vi "Quick Start - Complete Streaming with Datasource Creation.vi"() -> ()   [LabVIEW 2020]
uses:
  Nominal Client/Nominal Client.lvclass/Nominal Client.ctl
  8bc873d6-11f2-47b8-afa9-2ee06eb45ce7.vi
  Nominal Client/private_data.set.vi
  <vilib>/Utility/file.llb/Application Directory.vi
  <vilib>/Utility/error.llb/Error Cluster From Error Code.vi
  submodules/reqwest-labview/lv-src/reqwest/create.vi
  Nominal Client/Palette Items/who_am_i.vi
  Nominal Client/asset.get.vi
  User/User.lvclass
  Nominal Client/Nominal Client.lvclass
  nominal types/workspace/workspace.lvclass
  submodules/reqwest-labview/lv-src/reqwest/reqwest.lvclass
  asset/asset.lvclass
  datasources/dataset/dataset.lvclass
  submodules/nominal-streaming-labview-ffi/lv_src/Stream/Stream.lvclass
  submodules/nominal-streaming-labview-ffi/lv_src/Channel/Channel.lvclass
panel:
  in  "API Token":string
  in  "Stop":bool
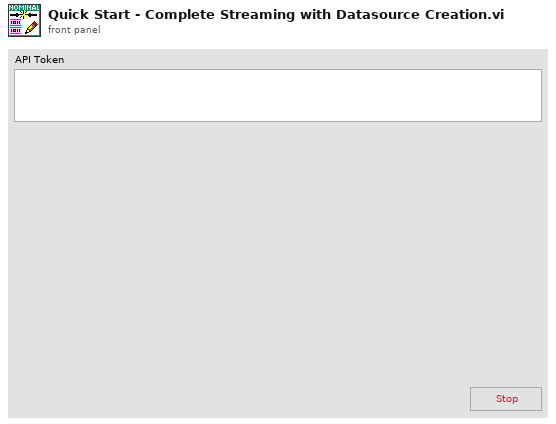
[diagram p1: front panel]
types:
  T1 = cluster{"channel":string, "current time":timestamp, "data":dbl}
  T2 = cluster{"[0]":refnum<queue>, "[1]":refnum<queue>, "[2]":refnum<queue>}
  T3 = cluster{"channel":string, "current time":timestamp, "data":dbl}[]
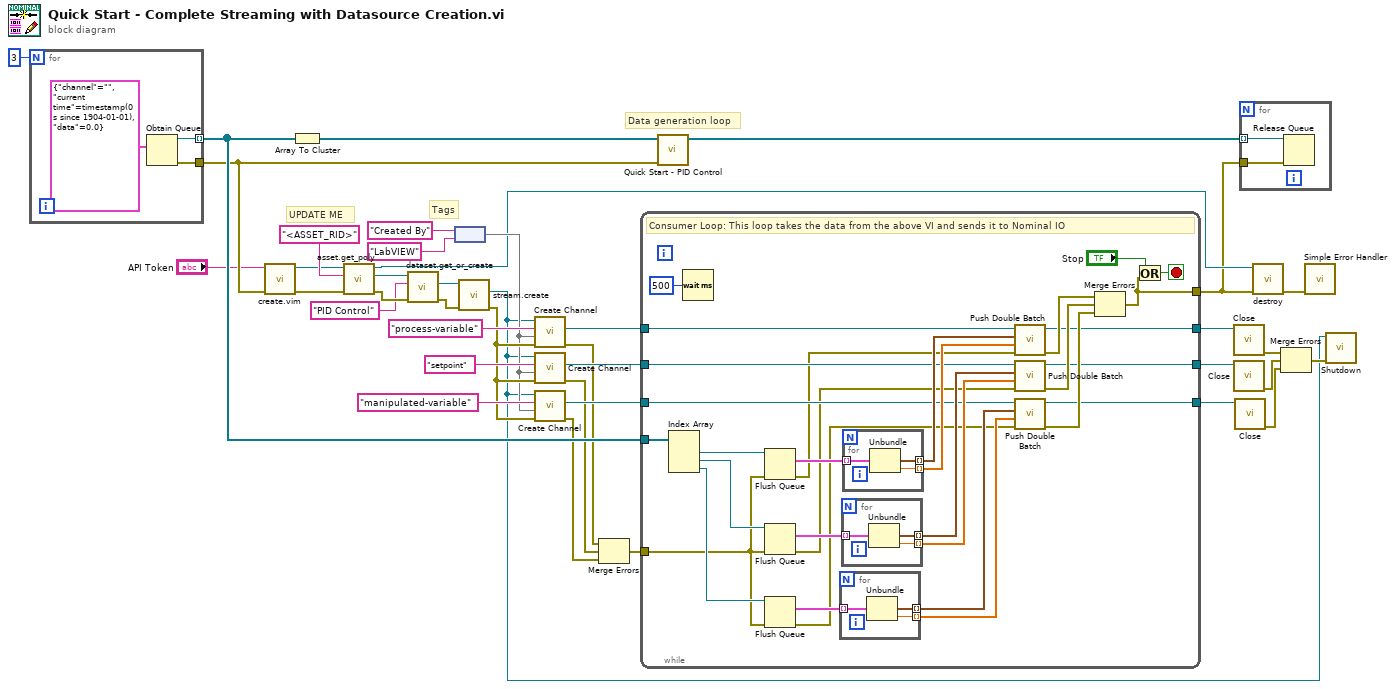
[diagram p0: block diagram]
diagram:
  # "UPDATE ME"
  # "Tags"
  # "Data generation loop"
  n1 = for {
    N: 3 -> [_]
    tunnel: [w40] -> w36 mode=indexing
    tunnel: [w39] -> w34
    n2 = Obtain Queue(element data type=T1 {"channel"="", "current time"=timestamp(0 s since 1904-01-01), "data"=0.0}) -> (queue out=w40:refnum<queue>, error out=w39:errorcluster)  [unwired: 4 in, 1 out]
  }
  n3 = call "create.vim"("error in"=w34, "API Token (string or path)"="API Token") -> ("error out"=w30:errorcluster, "Nominal Client"=w31:refnum<class "Nominal Client.lvclass">)  [unwired: 7 in, 1 out]
  n4 = Array To Cluster(array=w36) -> (cluster=w35:T2)
  n5 = call-poly "asset.get_poly.vi"("error in"=w30, "Asset RID"="<ASSET_RID>", "Nominal Client in"=w31) -> ("error out"=w28:errorcluster, "Asset"=w29:refnum<class "asset.lvclass">, "Nominal Client out"=w10:refnum<class "Nominal Client.lvclass">)  [unwired: 6 in]
  n6 = call "dataset.get_or_create.vi"("error in"=w28, "Datascope Name"="PID Control", "asset in"=w29) -> ("error out"=w25:errorcluster, "dataset"=w26:refnum<class "dataset.lvclass">)  [unwired: 6 in, 1 out]
  n7 = node("Created By", "LabVIEW") -> (w15:map{string, string})
  n8 = call "stream.create.vi"("error in (no error)"=w25, "dataset in"=w26) -> ("error out"=w18:errorcluster, "Stream"=w1:refnum<class "Stream.lvclass">)  [unwired: 7 in, 1 out]
  n9 = call "Create Channel.vi"("error in (no error)"=w18, "Tags"=w15, "Channel Name"="process-variable" ("String"), "Nominal Streaming in"=w1) -> ("error out"=w14:errorcluster, "Channel"=w24:refnum<class "Channel.lvclass">)  [unwired: 5 in, 1 out]
  n10 = call "Create Channel.vi"("error in (no error)"=w18, "Tags"=w15, "Channel Name"="setpoint" ("String"), "Nominal Streaming in"=w1) -> ("error out"=w13:errorcluster, "Channel"=w19:refnum<class "Channel.lvclass">)  [unwired: 5 in, 1 out]
  n11 = call "Create Channel.vi"("error in (no error)"=w18, "Tags"=w15, "Channel Name"="manipulated-variable" ("String"), "Nominal Streaming in"=w1) -> ("error out"=w12:errorcluster, "Channel"=w20:refnum<class "Channel.lvclass">)  [unwired: 5 in, 1 out]
  n12 = Merge Errors(w14, w13, w12) -> (w11:errorcluster)
  n13 = while {
    tunnel: w36 -> [w68]
    tunnel: w24 -> [w59]
    tunnel: w20 -> [w55]
    tunnel: w19 -> [w58]
    tunnel: w11 -> [w52]
    tunnel: [w45] -> w9
    tunnel: [w44] -> w8
    tunnel: [w43] -> w7
    tunnel: [w42] -> w6
    stop <- w70 stop-if-true
    # "Consumer Loop: This loop takes the data from the above VI and sends it to Nominal IO"
    n14 = Index Array(array=w68) -> (element #1=w67:refnum<queue>, element #2=w60:refnum<queue>, element #3=w56:refnum<queue>)  [unwired: 3 in]
    n15 = Wait (ms)(milliseconds to wait=u32 500) -> ()  [unwired: 1 out]
    n16 = Flush Queue(queue=w67, error in (no error)=w52) -> (remaining elements=w66:T3, error out=w51:errorcluster)  [unwired: 1 out]
    n17 = Flush Queue(queue=w60, error in (no error)=w52) -> (remaining elements=w61:T3, error out=w50:errorcluster)  [unwired: 1 out]
    n18 = Flush Queue(queue=w56, error in (no error)=w52) -> (remaining elements=w57:T3, error out=w49:errorcluster)  [unwired: 1 out]
    n19 = for {
      tunnel: w57 -> [w74] mode=indexing
      tunnel: [w72] -> w54 mode=indexing
      tunnel: [w73] -> w53 mode=indexing
      n20 = Unbundle(w74) -> ("current time"=w72:timestamp, "data"=w73:dbl)  [unwired: 1 out]
    }
    n21 = for {
      tunnel: w61 -> [w77] mode=indexing
      tunnel: [w75] -> w62 mode=indexing
      tunnel: [w76] -> w63 mode=indexing
      n22 = Unbundle(w77) -> ("current time"=w75:timestamp, "data"=w76:dbl)  [unwired: 1 out]
    }
    n23 = for {
      tunnel: w66 -> [w80] mode=indexing
      tunnel: [w78] -> w65 mode=indexing
      tunnel: [w79] -> w64 mode=indexing
      n24 = Unbundle(w80) -> ("current time"=w78:timestamp, "data"=w79:dbl)  [unwired: 1 out]
    }
    n25 = call "Push Double Batch.vi"("error in (no error)"=w51, "Values"=w64, "Timestamps"=w65, "Channel in"=w59) -> ("error out"=w48:errorcluster, "Channel out"=w44:refnum<class "Channel.lvclass">)  [unwired: 6 in]
    n26 = call "Push Double Batch.vi"("error in (no error)"=w50, "Values"=w63, "Timestamps"=w62, "Channel in"=w58) -> ("error out"=w47:errorcluster, "Channel out"=w43:refnum<class "Channel.lvclass">)  [unwired: 6 in]
    n27 = call "Push Double Batch.vi"("error in (no error)"=w49, "Values"=w53, "Timestamps"=w54, "Channel in"=w55) -> ("error out"=w46:errorcluster, "Channel out"=w42:refnum<class "Channel.lvclass">)  [unwired: 6 in]
    n28 = Merge Errors(w48, w47, w46) -> (w45:errorcluster)
    n29 = Or(x="Stop", y=w45) -> (x .or. y?=w70:bool)
  }
  n30 = call "Quick Start - PID Control.vi"("error in (no error)"=w34, "Data"=w35) -> ()  [unwired: 10 in]
  n31 = call "Close.vi"("Channel in"=w8) -> ("error out"=w3:errorcluster)  [unwired: 10 in]
  n32 = call "Close.vi"("Channel in"=w7) -> ("error out"=w4:errorcluster)  [unwired: 10 in]
  n33 = call "Close.vi"("Channel in"=w6) -> ("error out"=w5:errorcluster)  [unwired: 10 in]
  n34 = for {
    tunnel: w36 -> [w82] mode=indexing
    tunnel: w9 -> [w81]
    n35 = Release Queue(queue=w82, error in (no error)=w81) -> ()  [unwired: 1 in, 3 out]
  }
  n36 = call "destroy.vi"("error in"=w9, "Nominal Client"=w10) -> ("error out"=w38:errorcluster)  [unwired: 9 in]
  n37 = Merge Errors(w3, w4, w5) -> (w2:errorcluster)
  n38 = call <vilib>:"Simple Error Handler.vi"("error in (no error)"=w38) -> ()  [unwired: 4 in, 5 out]
  n39 = call "Shutdown.vi"("error in (no error)"=w2, "Nominal Streaming in"=w1) -> ()  [unwired: 8 in, 2 out]
